vi "Get Info.vi"(8 "error in (no error)":errorcluster, 11 "Channel Config in":refnum<class "Channel Config.lvclass">) -> (0 "error out":errorcluster, 2 "Info":T1, 3 "Channel Config out":refnum<class "Channel Config.lvclass">)   [LabVIEW 2020, in "Vecto.lvlib" / "Channel Config.lvclass"]
uses:
  Channel Config.lvclass
  Channel Info.ctl
  Vecto.lvlib
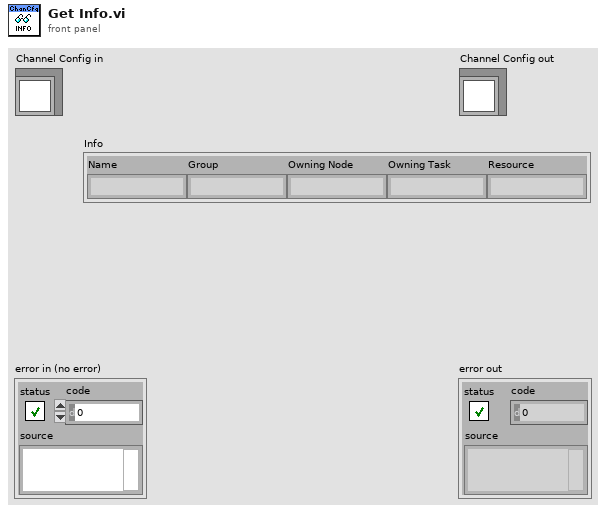
[diagram p1: front panel]
types:
  T1 = typedef "Vecto.lvlib/Channel Info.ctl" = cluster{"Name":string, "Group":string, "Owning Node":string, "Owning Task":string, "Resource":string}
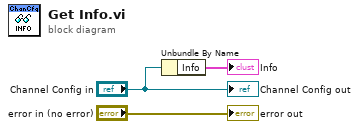
[diagram p0: block diagram]
diagram:
  n1 = Unbundle By Name("Channel Config in") -> ("Info"=→"Info":T1)
  "error out" <- "error in (no error)"
  "Channel Config out" <- "Channel Config in"
